vi "configureCamera.vi"(8 "error in (no error)":errorcluster, 9 "video":bool, 10 "device":string, 11 "AtomChipHWC in":refnum<class "AtomChipHWC.lvclass">) -> (0 "error out":errorcluster, 3 "AtomChipHWC out":refnum<class "AtomChipHWC.lvclass">)   [LabVIEW 2009, in "Hardware.lvlib" / "HWControllers.lvlib" / "AtomChipHWC.lvclass"]
uses:
  AtomChipHWC.lvclass
  AtomChipHWC.lvclass/AtomChipHWC.ctl
  Tools/Filing/FileSystem/FileSystem.lvclass
  Network Controllers/NetworkCamera/NetworkCamera.lvclass
  Tools/CameraSettings/CamaraSettings.lvclass
  HWController.lvclass
  Network Controllers/CameraNetworkController/CameraNetworkController.lvclass
  Tools/Filing/FileNeologist/FileNeologist.lvclass
  Tools/Filing.lvlib
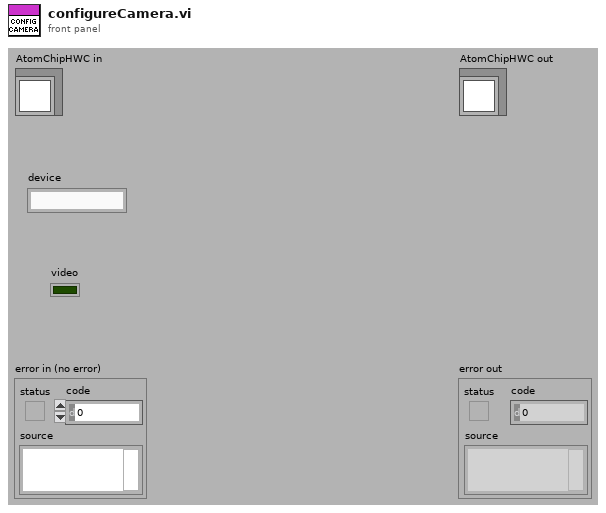
[diagram p1: front panel]
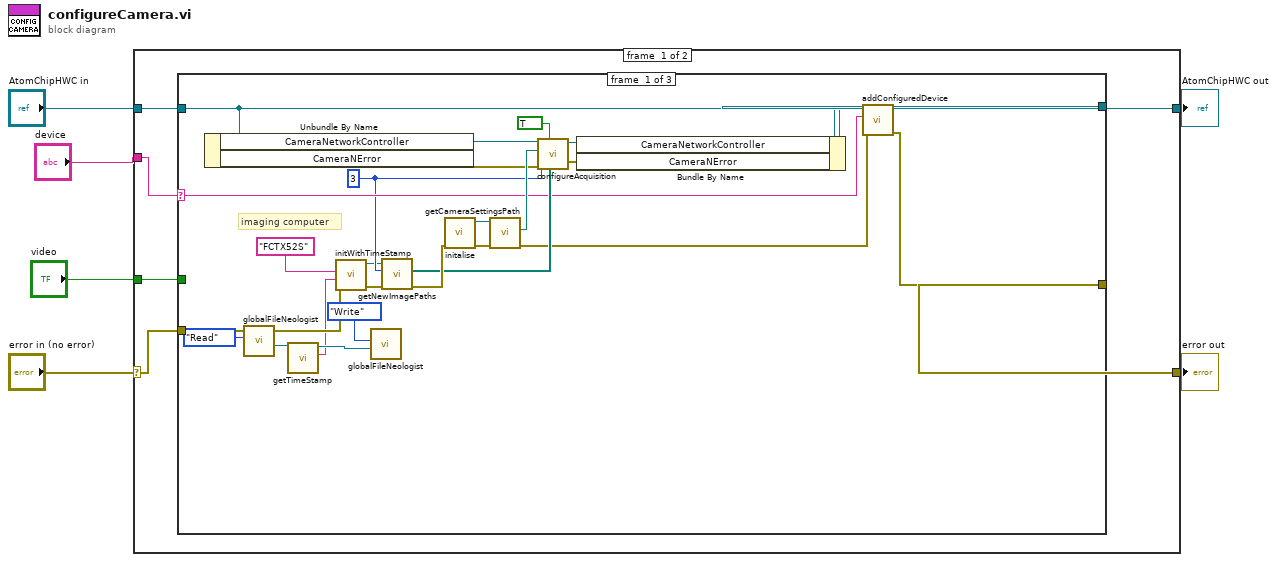
[diagram p0: block diagram]
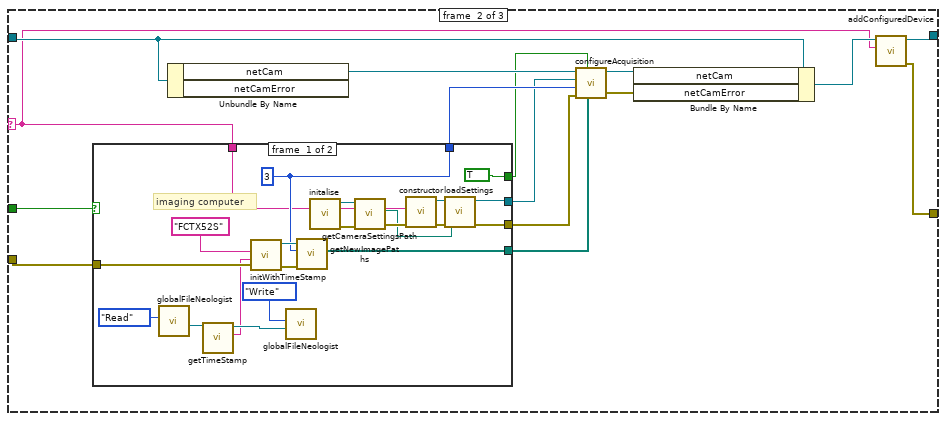
[diagram p2: hidden frame]
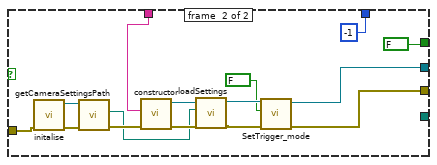
[diagram p3: hidden frame]
diagram:
  n1 = case shown="No Error" "error in (no error)" {
    selector: "error in (no error)" -> [w11 w93]
    tunnel: [w10 w93] -> w5
    tunnel: [w12 w92] -> w3
    tunnel: "AtomChipHWC in" -> [w9 w92]
    tunnel: "device" -> [w8 _]
    tunnel: "video" -> [w7 _]
    frame #0 {
      n2 = case shown="\"Pixelfly\", \"ProEM_WinX32\"" w8 {
        selector: w8 -> [w27 w43 _]
        tunnel: [w28 w51 w91] -> w12
        tunnel: w11 -> [w22 w49 w90]
        tunnel: [w26 w50 w90] -> w10
        tunnel: w9 -> [w37 w53 w91]
        tunnel: w7 -> [_ w39 _]
        frame #0 {
          w25 = 3
          # "imaging computer"
          n3 = Unbundle By Name(w37) -> ("CameraNetworkController"=w38:refnum<class "CameraNetworkController.lvclass">, "CameraNError"=w15:errorcluster)
          n4 = call "globalFileNeologist.vi"("Action"=enum16{"Write", "Read"}."Read") -> ("FileNeologist out"=w18:refnum<class "FileNeologist.lvclass">)  [unwired: 10 in]
          n5 = call "getTimeStamp.vi"("FileNeologist in"=w18) -> ("TimeStamp"=w16:string, "FileNeologist out"=w17:refnum<class "FileNeologist.lvclass">)  [unwired: 8 in, 1 out]
          n6 = call "initWithTimeStamp.vi"("error in (no error)"=w22, "timeStamp"=w16, "computer name"="FCTX52S") -> ("error out"=w24:errorcluster, "FileNeologist out"=w23:refnum<class "FileNeologist.lvclass">)  [unwired: 7 in]
          n7 = call "globalFileNeologist.vi"("FileNeologist in"=w17, "Action"=enum16{"Write", "Read"}."Write") -> ()  [unwired: 9 in, 1 out]
          n8 = call "getNewImagePaths.vi"("error in (no error)"=w24, "numberOfImages"=w25, "FileNeologist in"=w23) -> ("error out"=w31:errorcluster, "Paths"=w30:path[])  [unwired: 6 in, 1 out]
          n9 = call "initalise.vi"("error in (no error)"=w31) -> ("error out"=w33:errorcluster, "FileSystem out"=w34:refnum<class "FileSystem.lvclass">)  [unwired: 9 in]
          n10 = call-dynamic "getCameraSettingsPath.vi"("error in (no error)"=w33, "FileSystem.lvclass in"=w34) -> ("error out"=w13:errorcluster, "CameraSettingsPath"=w32:path)  [unwired: 7 in, 1 out]
          n11 = call "configureAcquisition.vi"("imagePaths"=w30, "save?"=TRUE, "error in (no error)"=w15, "numberImages"=w25, "settingsPath"=w32, "CameraNetworkController in"=w38) -> ("error out"=w14:errorcluster, "CameraNetworkController out"=w36:refnum<class "CameraNetworkController.lvclass">)  [unwired: 4 in]
          n12 = Bundle By Name(cluster=w37, "CameraNetworkController"=w36, "CameraNError"=w14) -> (w29:refnum<class "AtomChipHWC.lvclass">)
          n13 = call "addConfiguredDevice.vi"("error in (no error)"=w13, "deviceName"=w27, "HWController in"=w29) -> ("error out"=w26:errorcluster, "HWController out"=w28:refnum<class "AtomChipHWC.lvclass">)  [unwired: 7 in]
        }
        frame #1 {
          n14 = case shown="True" w39 {
            tunnel: w49 -> [w70 w80]
            tunnel: [w63 -1] -> w46
            tunnel: [w62 _] -> w44
            tunnel: w43 -> [w57 w82]
            tunnel: [w56 w77] -> w42
            tunnel: [w55 w76] -> w41
            tunnel: [TRUE FALSE] -> w40
            frame #0 {
              w63 = 3
              # "imaging computer"
              n15 = call "globalFileNeologist.vi"("Action"=enum16{"Write", "Read"}."Read") -> ("FileNeologist out"=w66:refnum<class "FileNeologist.lvclass">)  [unwired: 10 in]
              n16 = call "getTimeStamp.vi"("FileNeologist in"=w66) -> ("TimeStamp"=w64:string, "FileNeologist out"=w65:refnum<class "FileNeologist.lvclass">)  [unwired: 8 in, 1 out]
              n17 = call "initWithTimeStamp.vi"("error in (no error)"=w70, "timeStamp"=w64, "computer name"="FCTX52S") -> ("error out"=w72:errorcluster, "FileNeologist out"=w71:refnum<class "FileNeologist.lvclass">)  [unwired: 7 in]
              n18 = call "globalFileNeologist.vi"("FileNeologist in"=w65, "Action"=enum16{"Write", "Read"}."Write") -> ()  [unwired: 9 in, 1 out]
              n19 = call "getNewImagePaths.vi"("error in (no error)"=w72, "numberOfImages"=w63, "FileNeologist in"=w71) -> ("Paths"=w62:path[])  [unwired: 6 in, 2 out]
              n20 = call "initalise.vi"() -> ("error out"=w73:errorcluster, "FileSystem out"=w74:refnum<class "FileSystem.lvclass">)  [unwired: 10 in]
              n21 = call-dynamic "getCameraSettingsPath.vi"("error in (no error)"=w73, "FileSystem.lvclass in"=w74) -> ("error out"=w60:errorcluster, "CameraSettingsPath"=w59:path)  [unwired: 7 in, 1 out]
              n22 = call "constructor.vi"("error in (no error)"=w60, "camera settings"=w57) -> ("error out"=w58:errorcluster, "CamaraSettings out"=w61:refnum<class "CamaraSettings.lvclass">)  [unwired: 8 in]
              n23 = call-dynamic "loadSettings.vi"("error in (no error)"=w58, "Path"=w59, "CamaraSettings in"=w61) -> ("error out"=w55:errorcluster, "CamaraSettings out"=w56:refnum<class "CamaraSettings.lvclass">)  [unwired: 7 in]
            }
            frame #1 {
              n24 = call "initalise.vi"("error in (no error)"=w80) -> ("error out"=w86:errorcluster, "FileSystem out"=w87:refnum<class "FileSystem.lvclass">)  [unwired: 9 in]
              n25 = call-dynamic "getCameraSettingsPath.vi"("error in (no error)"=w86, "FileSystem.lvclass in"=w87) -> ("error out"=w84:errorcluster, "CameraSettingsPath"=w81:path)  [unwired: 7 in, 1 out]
              n26 = call "constructor.vi"("error in (no error)"=w84, "camera settings"=w82) -> ("error out"=w83:errorcluster, "CamaraSettings out"=w85:refnum<class "CamaraSettings.lvclass">)  [unwired: 8 in]
              n27 = call-dynamic "loadSettings.vi"("error in (no error)"=w83, "Path"=w81, "CamaraSettings in"=w85) -> ("error out"=w78:errorcluster, "CamaraSettings out"=w79:refnum<class "CamaraSettings.lvclass">)  [unwired: 7 in]
              n28 = call-dynamic "SetTrigger_mode.vi"("error in (no error)"=w78, "trigger_mode"=FALSE, "CamaraSettings in"=w79) -> ("error out"=w76:errorcluster, "CamaraSettings out"=w77:refnum<class "CamaraSettings.lvclass">)  [unwired: 7 in]
            }
          }
          n29 = Unbundle By Name(w53) -> ("netCam"=w48:refnum<class "NetworkCamera.lvclass">)  [unwired: 1 out]
          n30 = call-dynamic "configureAcquisition.vi"("imagePaths"=w44, "saveImages?"=w40, "error in (no error)"=w41, "number of Images"=w46, "CamaraSettings"=w42, "NetworkCamera in"=w48) -> ("error out"=w45:errorcluster, "NetworkCamera out"=w47:refnum<class "NetworkCamera.lvclass">)  [unwired: 4 in]
          n31 = Bundle By Name(cluster=w53, "netCam"=w47, "netCamError"=w45) -> (w52:refnum<class "AtomChipHWC.lvclass">)
          n32 = call "addConfiguredDevice.vi"("deviceName"=w43, "HWController in"=w52) -> ("error out"=w50:errorcluster, "HWController out"=w51:refnum<class "AtomChipHWC.lvclass">)  [unwired: 8 in]
        }
        frame #2 {
        }
      }
    }
    frame #1 {
    }
  }
  "error out" <- w5
  "AtomChipHWC out" <- w3
